vi "ReadBatteryVoltage.vi"(11 "Queue in":refnum<queue>) -> (0 "error out":errorcluster, 3 "B/AI0 (Pin 3) [volts]":dbl(knob) scale=0.0..5.0)   [LabVIEW 2013]
doc: "Reads the battery sensor through an analog pin off the MyRIO. Needs to be calibrated to the voltage divider.\n\nEric Schneider, March 2014"
uses:
  <vilib>/myRIO/Instrument Drivers/Onboard IO/AI/vis/Smart Open.vi
  <vilib>/myRIO/Instrument Drivers/Onboard IO/AI/vis/Read.vi
  <vilib>/myRIO/Instrument Drivers/Onboard IO/AI/vis/Open.vi
  <vilib>/myRIO/Common/Instrument Driver Framework/myRIO v1.0/AI/vis/myRIO v1.1 Open AI.vi
  <vilib>/myRIO/Common/Instrument Driver Framework/Utilities/vis/Validate Channels.vi
  <vilib>/myRIO/Common/Instrument Driver Framework/myRIO v1.0/AI/vis/myRIO v1.0 Reserve AI.vi
  <vilib>/myRIO/Common/Instrument Driver Framework/myRIO v1.0/AI/vis/myRIO v1.0 Build MUX Configuration AI.vi
  <vilib>/myRIO/Common/Instrument Driver Framework/myRIO v1.0/Resource Manager/vis/myRIO v1.0 Reserve Channel List.vi
  <vilib>/myRIO/Common/Instrument Driver Framework/myRIO v1.0/Resource Manager/vis/myRIO v1.0 Reserve Channel.vi
  <vilib>/myRIO/Common/Instrument Driver Framework/myRIO v1.0/Resource Manager/vis/myRIO v1.0 Unreserve Channel.vi
  <vilib>/myRIO/Common/Instrument Driver Framework/myRIO v1.0/Resource Manager/vis/myRIO v1.0 Build Mutex Name.vi
  <vilib>/myRIO/Common/Instrument Driver Framework/myRIO v1.0/myRIO v1.1 Open.vi
  <vilib>/myRIO/Common/Instrument Driver Framework/myRIO v1.0/AI/vis/myRIO v1.0 Get Scaling Constants AI.vi
  <vilib>/Utility/VariantDataType/GetNumericInfo.vi
  <vilib>/Utility/error.llb/Error Cluster From Error Code.vi
  <vilib>/myRIO/Common/Instrument Driver Framework/Utilities/vis/IO Manager.vi
  <vilib>/myRIO/Common/Instrument Driver Framework/Utilities/vis/Configuration Manager.vi
  <vilib>/myRIO/Common/Instrument Driver Framework/myRIO v1.0/myRIO v1.0 Close.vi
  <vilib>/myRIO/Common/Instrument Driver Framework/myRIO v1.0/AI/vis/myRIO v1.0 Read AI.vi
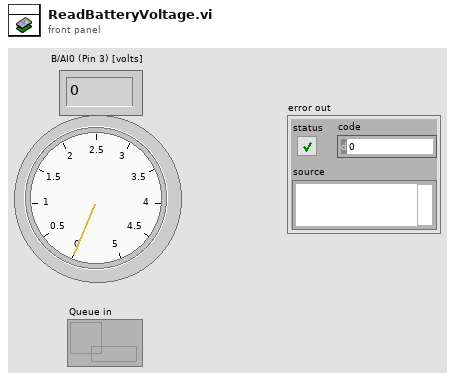
[diagram p1: front panel]
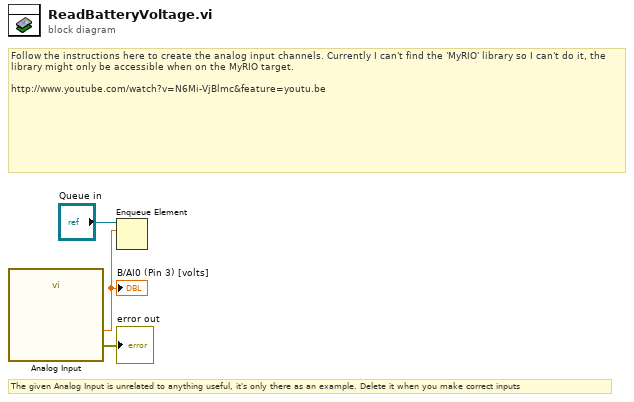
[diagram p0: block diagram]
diagram:
  # "The given Analog Input is unrelated to anything useful, it's only there as an example. Delete it when you make correct inputs"
  # "Follow the instructions here to create the analog input channels. Currently I can't find the 'MyRIO' library so I can't do it, the library might only be accessible when on the MyRIO target.\n\nhttp://www.youtube.com/watch?v=N6Mi-VjBlmc&feature=youtu.be"
  n1 = call "Analog Input"() -> ("B/AI0 (Pin 3)"=w1:dbl, "error out"=→"error out":errorcluster)  [unwired: 26 in]
  "B/AI0 (Pin 3) [volts]" <- w1
  n2 = Enqueue Element(queue="Queue in", element=w1) -> ()  [unwired: 2 in, 3 out]
